vi "Imaging_clock.vi"(8 "FPGA Cycle Counters XY":T1, 9 "FPGA Cycle Parameters XY":T3={"FPGA Cycle Parameters X"={"Imaging cycles"=285714, "Settling cycles"=71429, "Resting cycles"=42857, "Phase advance per cycle"=0.0001399517059326172, "Imaging Multiplier advance per cycle"=0.00286865234375, "Settling Multiplier advance per cycle"=-0.0057373046875, "Imaging Initial Multiplier"=0.0, "Initial Phase"=0.0}, "FPGA Cycle Parameters Y"={"Imaging cycles"=285714, "Settling cycles"=71429, "Resting cycles"=42857, "Phase advance per cycle"=0.0001399517059326172, "Imaging Multiplier advance per cycle"=0.00286865234375, "Settling Multiplier advance per cycle"=-0.0057373046875, "Imaging Initial Multiplier"=0.0, "Initial Phase"=0.0}}) -> (3 "Imaging Clock Out":bool)   [LabVIEW 2010]
uses:
  FPGA_Typedefs/FPGA Cycle Parameters XY.ctl
  FPGA_Typedefs/FPGA Cycle Parameters.ctl
  FPGA_Typedefs/FPGA Cycle Counters XY.ctl
  FPGA_Typedefs/FPGA Cycle Counters.ctl
  <vilib>/eio/EIONode/EIONode.xnode
  <vilib>/rvi/eio/nirviEIOImplementation/nirviEIOImplementation.xnode
  <vilib>/rvi/eio/common/nirviEmuClasses.ctl
  <vilib>/rvi/eio/common/nirviEmuTemplateMethod_noerrors.vi
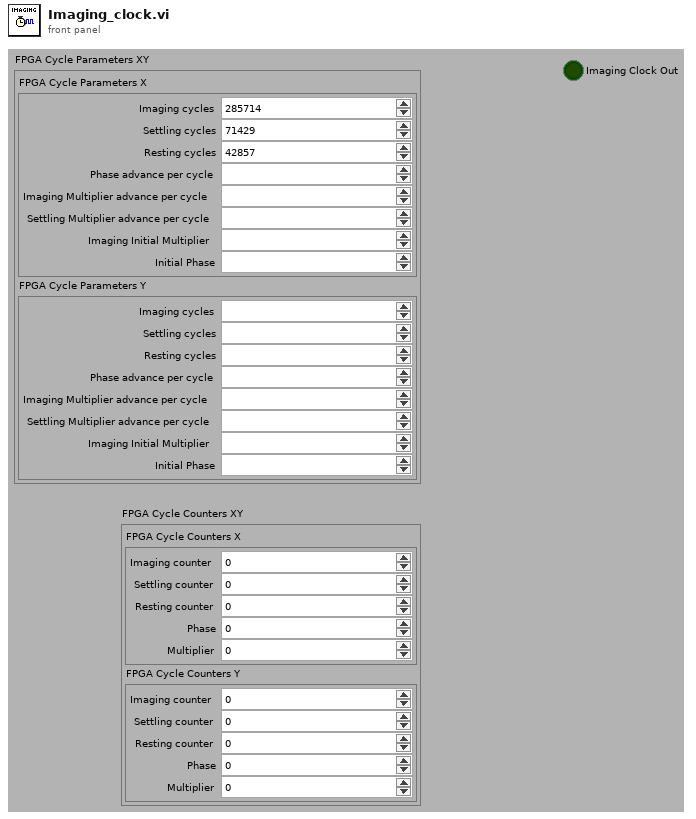
[diagram p1: front panel]
types:
  T1 = typedef "FPGA Cycle Counters XY.ctl" = cluster{"FPGA Cycle Counters X":T2, "FPGA Cycle Counters Y":T2}
  T2 = typedef "FPGA Cycle Counters.ctl" = cluster{"Imaging counter":i32, "Settling counter":i32, "Resting counter":i32, "Phase":fxp<+,32,1>, "Multiplier":fxp<+/-,43,12>}
  T3 = typedef "FPGA Cycle Parameters XY.ctl" = cluster{"FPGA Cycle Parameters X":T4, "FPGA Cycle Parameters Y":T4}
  T4 = typedef "FPGA Cycle Parameters.ctl" = cluster{"Imaging cycles":i32, "Settling cycles":i32, "Resting cycles":i32, "Phase advance per cycle":fxp<+,32,0>, "Imaging Multiplier advance per cycle":fxp<+/-,32,0>, "Settling Multiplier advance per cycle":fxp<+/-,32,0>, "Imaging Initial Multiplier":fxp<+/-,43,12>, "Initial Phase":fxp<+,32,1>}
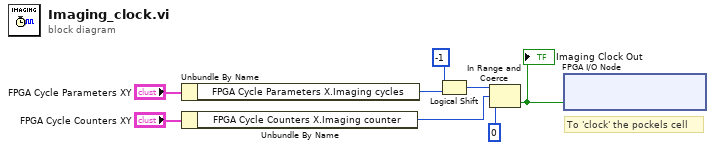
[diagram p0: block diagram]
diagram:
  # "To 'clock' the pockels cell"
  n1 = Unbundle By Name("FPGA Cycle Parameters XY") -> ("FPGA Cycle Parameters X.Imaging cycles"=w6:i32)
  n2 = Unbundle By Name("FPGA Cycle Counters XY") -> ("FPGA Cycle Counters X.Imaging counter"=w3:i32)
  n3 = Logical Shift(y=i8 -1, x=w6) -> (x << y=w4:i32)
  n4 = In Range and Coerce(upper limit=w4, x=w3, lower limit=u32 0) -> (In Range?=w1:bool)  [unwired: 1 out]
  "Imaging Clock Out" <- w1
  n5 = xnode "FPGA I/O Node"("Connector0/DIO30"=w1) -> ()  [unwired: 1 in, 1 out]
